vi "login_popup.vi"(8 "Error In":errorcluster) -> (0 "Error Out":errorcluster)   [LabVIEW 2013, in "main.lvlib"]
uses:
  main.lvlib
  <userlib>/_MGI/Error Handling/MGI Suppress Error Code/MGI Suppress Error Code (Scalar).vi
panel:
  in  "LoginCancelBtn":bool
  in  "LoginBtn":bool
  in  "Password":string
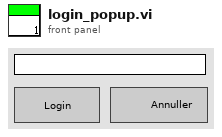
[diagram p1: front panel]
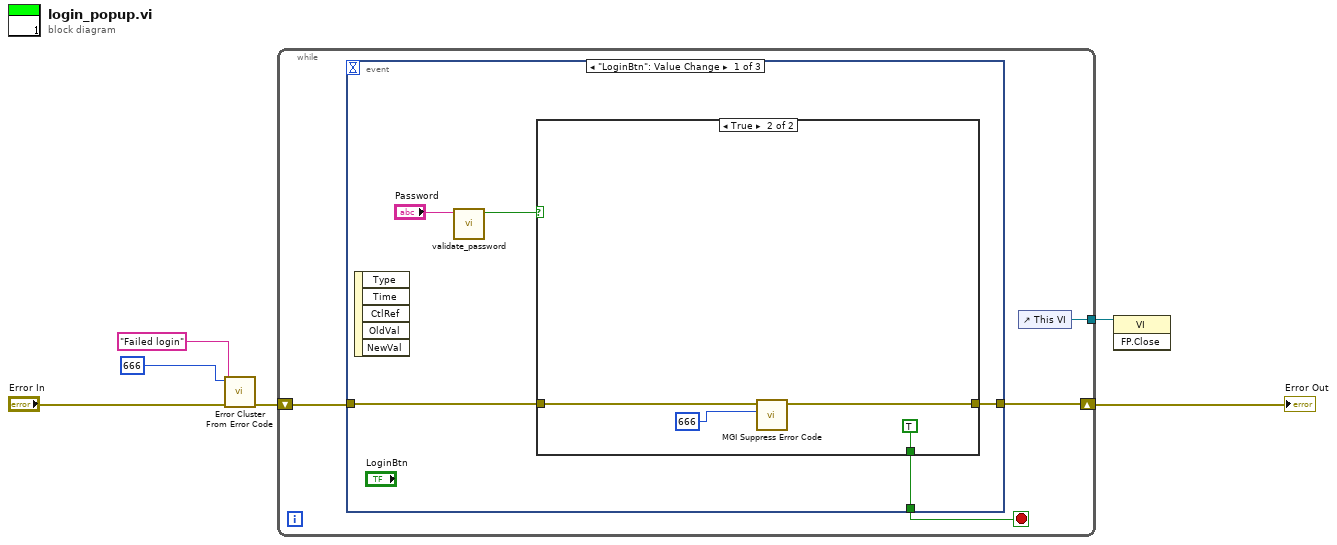
[diagram p0: block diagram]
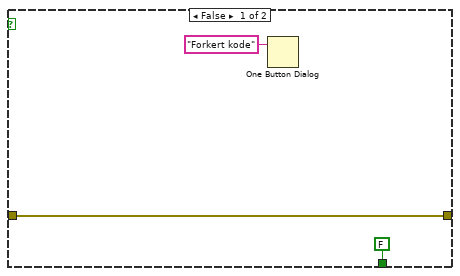
[diagram p2: hidden frame]
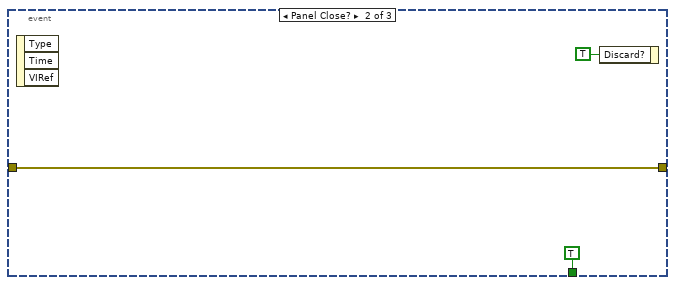
[diagram p3: hidden frame]
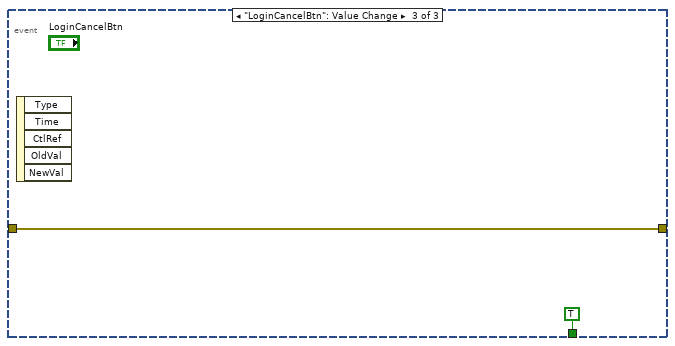
[diagram p4: hidden frame]
diagram:
  n1 = call <vilib>:"Error Cluster From Error Code.vi"("error in (no error)"="Error In", "error message (\"\")"="Failed login" ("error message (\"\")"), "error code (0)"=666) -> ("error out"=w3:errorcluster)  [unwired: 6 in]
  n2 = while {
    shift-right: [w9] -> w2
    shift-left: w3 -> [w8]
    tunnel: [w7] -> w1
    stop <- w10 stop-if-true
    n3 = event shown="[0] \"LoginBtn\": Value Change" {
      selector: _ -> [_ _ _]
      dyn-events: _ -> [_ _ _]
      timeout: _ -> [_ _ _]
      tunnel: [w13 TRUE TRUE] -> w10
      tunnel: w8 -> [w12 w24 w27]
      tunnel: [w11 w24 w27] -> w9
      event "LoginBtn": Value Change {
        n4 = event-data() -> ()  [unwired: 1 in, 5 out]
        n5 = call "validate_password.vi"("Password"="Password") -> ("Accept"=w14:bool)  [unwired: 10 in]
        n6 = case shown="True" w14 {
          tunnel: [FALSE TRUE] -> w13
          tunnel: w12 -> [w16 w20]
          tunnel: [w16 w21] -> w11
          frame False {
            n7 = One Button Dialog(message="Forkert kode") -> ()  [unwired: 1 in, 1 out]
          }
          frame True {
            n8 = call-poly <userlib>:"MGI Suppress Error Code.vi"("Error Code"=666, "Error In"=w20) -> ("Error Out"=w21:errorcluster)  [unwired: 4 in, 1 out]
          }
        }
      }
      event Panel Close? {
        n9 = event-data() -> ()  [unwired: 1 in, 3 out]
        n10 = event-data("Discard?"=TRUE) -> ()  [unwired: 1 in, 1 out]
      }
      event "LoginCancelBtn": Value Change {
        n11 = event-data() -> ()  [unwired: 1 in, 5 out]
      }
    }
    n12 = control-ref of="This VI"() -> (w7:refnum<vi>)
  }
  "Error Out" <- w2
  n13 = invoke class="VI" method="FP.Close"(reference=w1) -> ()  [unwired: 2 in, 3 out]
